vi "DB_WriteInGen6.vi"(8 "error in (no error)":errorcluster, 9 "Equipo_Medicion":T2, 10 "PM_out":T1={"Equipo_Medicion"={"ID_EQUIPO"=0, "IP_EQUIPO"="", "NOMBRE_EQUIPO"="", "ESTADO_EQUIPO"="", "DESCRIPCION"="", "ID_MEDICION"=0, "ESTADO_MEDICION"="", "TIEMPO_MEDICION"="12-02-2019 18:41"}, "VIF_cluster"={"VL_VL"={"V1_V2"=0.0, "V2_V3"=0.0, "V3_V1"=0.0, "Avg_VL_VL"=0.0}, "IL_IL"={"I1"=0.0, "I2"=0.0, "I3"=0.0, "Avg_Amps"=0.0}, "Frecuency"=0.0, "Avg_Frecuency"=0.0}, "Power_cluster"={"Real Power (kW)"={"L1_kW"=0.0, "L2_kW"=0.0, "L3_kW"=0.0, "Total_kW"=0.0}, "Reactive Power (kVAR)"={"L1_kVAR"=0.0, "L2_kVAR"=0.0, "L3_kVAR"=0.0, "Total_kVAR"=0.0}, "Aparent Power (kVA)"={"L1_kVA"=0.0, "L2_kVA"=0.0, "L3_kVA"=0.0, "Total_kVA"=0.0}, "Power Factor (%)"={"L1_PF"=0.0, "L2_PF"=0.0, "L3_PF"=0.0, "Total_PF"=0.0}}, "THD_cluster"={"V_THD"={"V1_V2_THD"=0.0, "V2_V3_THD"=0.0, "V3_V1_THD"=0.0, "Avg_V_V_THD"=0.0}, "I_THD"={"I1_THD"=0.0, "I2_THD"=0.0, "I3_THD"=0.0, "I4_THD"=0.0, "Avg_I_THD"=0.0}}, "Polar_cluster"={"V_polar"={"V1_ang"=0.0, "V1_mag"=0.0, "V2_ang"=0.0, "V2_mag"=0.0, "V3_ang"=0.0, "V3_mag"=0.0}, "I_polar"={"I1_ang"=0.0, "I1_mag"=0.0, "I2_ang"=0.0, "I2_mag"=0.0, "I3_ang"=0.0, "I3_mag"=0.0}}}, 11 "DB in":T7) -> (0 "error out":errorcluster, 3 "closeDB":T7[](array[typedef]))   [LabVIEW 2018]
uses:
  <vilib>/addons/database/Connection.llb/Conn ObjectReference.ctl
  Controls/Equipos_Medicion_cluster.ctl
  Controls/Cluster_Data.ctl
  Controls/VIF_cluster.ctl
  Controls/Power_cluster.ctl
  Controls/THD_cluster.ctl
  Controls/Polar_cluster.ctl
  <vilib>/addons/database/NI_Database_API.lvlib
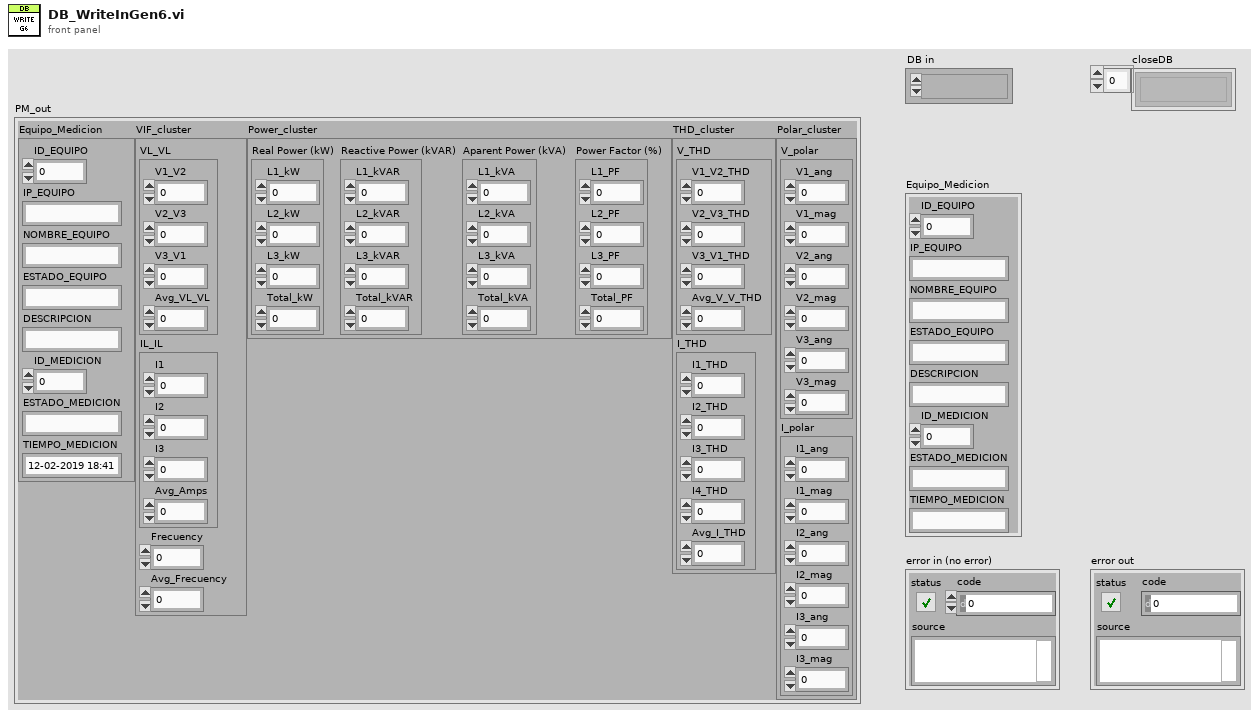
[diagram p1: front panel]
types:
  T1 = typedef "Cluster_Data.ctl" = cluster{"Equipo_Medicion":T2, "VIF_cluster":T3, "Power_cluster":T4, "THD_cluster":T5, "Polar_cluster":T6}
  T2 = typedef "Equipos_Medicion_cluster.ctl" = cluster{"ID_EQUIPO":i32, "IP_EQUIPO":string, "NOMBRE_EQUIPO":string, "ESTADO_EQUIPO":string, "DESCRIPCION":string, "ID_MEDICION":i32, "ESTADO_MEDICION":string, "TIEMPO_MEDICION":string}
  T3 = typedef "VIF_cluster.ctl" = cluster{"VL_VL":cluster{"V1_V2":sgl, "V2_V3":sgl, "V3_V1":sgl, "Avg_VL_VL":sgl}, "IL_IL":cluster{"I1":sgl, "I2":sgl, "I3":sgl, "Avg_Amps":sgl}, "Frecuency":sgl, "Avg_Frecuency":sgl}
  T4 = typedef "Power_cluster.ctl" = cluster{"Real Power (kW)":cluster{"L1_kW":sgl, "L2_kW":sgl, "L3_kW":sgl, "Total_kW":sgl}, "Reactive Power (kVAR)":cluster{"L1_kVAR":sgl, "L2_kVAR":sgl, "L3_kVAR":sgl, "Total_kVAR":sgl}, "Aparent Power (kVA)":cluster{"L1_kVA":sgl, "L2_kVA":sgl, "L3_kVA":sgl, "Total_kVA":sgl}, "Power Factor (%)":cluster{"L1_PF":sgl, "L2_PF":sgl, "L3_PF":sgl, "Total_PF":sgl}}
  T5 = typedef "THD_cluster.ctl" = cluster{"V_THD":cluster{"V1_V2_THD":sgl, "V2_V3_THD":sgl, "V3_V1_THD":sgl, "Avg_V_V_THD":sgl}, "I_THD":cluster{"I1_THD":sgl, "I2_THD":sgl, "I3_THD":sgl, "I4_THD":sgl, "Avg_I_THD":sgl}}
  T6 = typedef "Polar_cluster.ctl" = cluster{"V_polar":cluster{"V1_ang":sgl, "V1_mag":sgl, "V2_ang":sgl, "V2_mag":sgl, "V3_ang":sgl, "V3_mag":sgl}, "I_polar":cluster{"I1_ang":sgl, "I1_mag":sgl, "I2_ang":sgl, "I2_mag":sgl, "I3_ang":sgl, "I3_mag":sgl}}
  T7 = typedef "NI_Database_API.lvlib/Conn ObjectReference.ctl" = refnum<k1>
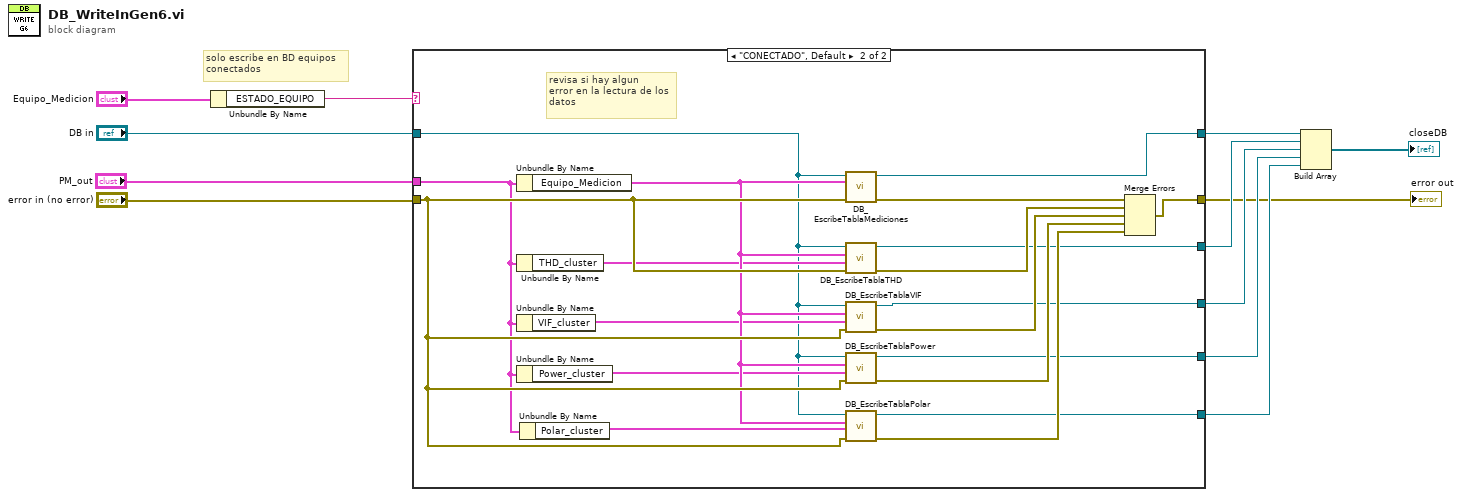
[diagram p0: block diagram]
diagram:
  # "solo escribe en BD equipos\nconectados"
  n1 = Unbundle By Name("Equipo_Medicion") -> ("ESTADO_EQUIPO"=w5:string)
  n2 = case shown="\"CONECTADO\", Default" w5 {
    tunnel: "error in (no error)" -> [w14 w33]
    tunnel: "DB in" -> [w13 w15]
    tunnel: [w14 w32] -> w2
    tunnel: [w13 w21] -> w7
    tunnel: [_ w20] -> w11
    tunnel: [_ w19] -> w10
    tunnel: [_ w18] -> w9
    tunnel: [_ w17] -> w8
    tunnel: "PM_out" -> [_ w16]
    frame "DESCONECTADO" {
      # "Equipo está deconectado"
    }
    frame "CONECTADO", Default {
      # "revisa si hay algun \nerror en la lectura de los\ndatos"
      n3 = Unbundle By Name(w16) -> ("Equipo_Medicion"=w31:T2)
      n4 = Unbundle By Name(w16) -> ("THD_cluster"=w30:T5)
      n5 = Unbundle By Name(w16) -> ("VIF_cluster"=w29:T3)
      n6 = Unbundle By Name(w16) -> ("Power_cluster"=w28:T4)
      n7 = Unbundle By Name(w16) -> ("Polar_cluster"=w27:T6)
      n8 = call "DB_EscribeTablaMediciones.vi"("error in (no error)"=w33, "Equipo_Medicion in"=w31, "db in"=w15) -> ("error out"=w26:errorcluster, "db out"=w21:T7)  [unwired: 7 in]
      n9 = call "DB_EscribeTablaTHD.vi"("error in (no error)"=w33, "THD_cluster"=w30, "Equipo_Medicion"=w31, "db in"=w15) -> ("error out"=w25:errorcluster, "db out"=w17:T7)  [unwired: 6 in]
      n10 = call "DB_EscribeTablaVIF.vi"("error in (no error)"=w33, "VIF_cluster"=w29, "Equipo_Medicion"=w31, "db in"=w15) -> ("error out"=w24:errorcluster, "db out"=w18:T7)  [unwired: 6 in]
      n11 = call "DB_EscribeTablaPower.vi"("error in (no error)"=w33, "Power_cluster"=w28, "Equipo_Medicion"=w31, "db in"=w15) -> ("error out"=w23:errorcluster, "db out"=w19:T7)  [unwired: 6 in]
      n12 = call "DB_EscribeTablaPolar.vi"("error in (no error)"=w33, "Polar_cluster"=w27, "Equipo_Medicion"=w31, "db in"=w15) -> ("error out"=w22:errorcluster, "db out"=w20:T7)  [unwired: 6 in]
      n13 = Merge Errors(w26, w25, w24, w23, w22) -> (w32:errorcluster)
    }
  }
  "error out" <- w2
  n14 = Build Array(w7, w8, w9, w10, w11) -> (→"closeDB":T7[])
